vi "send_array_2.vi"() -> ()   [LabVIEW 2013]
uses:
  <vilib>/Analysis/1siggen.llb/Ramp Pattern by Samples.vi
  <vilib>/Analysis/NI_AALBase.lvlib
panel:
  in  "elemszam":u16
  out "error out":errorcluster
  out "VISA resource name out":refnum<visa-resource-name>
  in  "VISA resource name 3":refnum<visa-resource-name>
  in  "error in (no error) 3":errorcluster
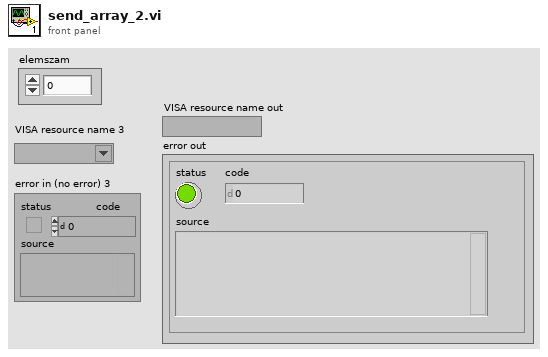
[diagram p1: front panel]
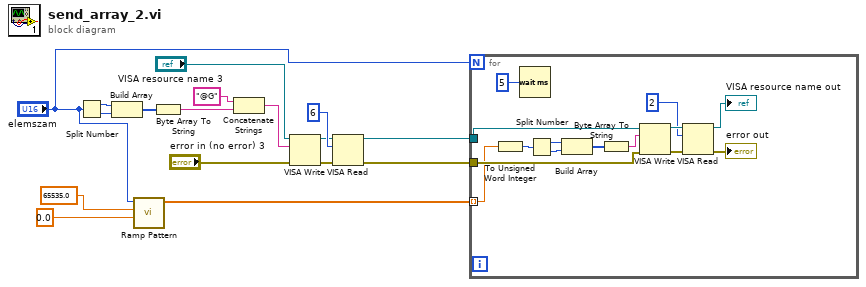
[diagram p0: block diagram]
diagram:
  n1 = Split Number(x="elemszam") -> (hi(x)=w10:u8, lo(x)=w9:u8)
  n2 = Build Array(w10, w9) -> (w8:u8[])
  n3 = call-poly <vilib>:"Ramp Pattern.vi"("start"=0.0, "end"=65535.0, "samples"="elemszam") -> ("Ramp Pattern"=w2:dbl[])  [unwired: 7 in, 1 out]
  n4 = Byte Array To String(unsigned byte array=w8) -> (string=w7:string)
  n5 = Concatenate Strings("@G" ("write buffer"), w7) -> (w14:string)
  n6 = VISA Write(VISA resource name="VISA resource name 3", write buffer=w14, error in (no error)="error in (no error) 3") -> (VISA resource name out=w12:refnum<visa-resource-name>, error out=w11:errorcluster)  [unwired: 1 out]
  n7 = VISA Read(VISA resource name=w12, byte count=u32 6, error in (no error)=w11) -> (VISA resource name out=w3:refnum<visa-resource-name>, error out=w4:errorcluster)  [unwired: 2 out]
  n8 = for {
    N: "elemszam" -> [_]
    tunnel: w2 -> [w24] mode=indexing
    tunnel: w4 -> [w30]
    tunnel: w3 -> [w29]
    n9 = To Unsigned Word Integer(number=w24) -> (unsigned 16bit integer=w27:u16)
    n10 = Wait (ms)(milliseconds to wait=u32 5) -> ()  [unwired: 1 out]
    n11 = Split Number(x=w27) -> (hi(x)=w25:u8, lo(x)=w26:u8)
    n12 = Build Array(w25, w26) -> (w28:u8[])
    n13 = Byte Array To String(unsigned byte array=w28) -> (string=w23:string)
    n14 = VISA Write(VISA resource name=w29, write buffer=w23, error in (no error)=w30) -> (VISA resource name out=w22:refnum<visa-resource-name>, error out=w31:errorcluster)  [unwired: 1 out]
    n15 = VISA Read(VISA resource name=w22, byte count=u32 2, error in (no error)=w31) -> (VISA resource name out=→"VISA resource name out":refnum<visa-resource-name>, error out=→"error out":errorcluster)  [unwired: 2 out]
  }
